vi "FTW-StressTest-Endpoint-CreateDestroy.vi"() -> ()   [LabVIEW 2012]
uses:
  src/Socket/FTW-Socket-Type.ctl
  src/Endpoint/FTW-Endpoint.lvclass
panel:
  out "x*y":i32
  out "error out":errorcluster
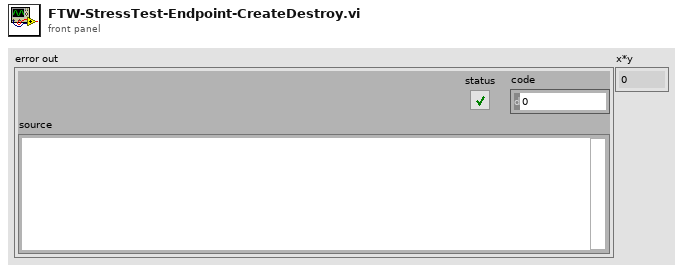
[diagram p1: front panel]
types:
  T1 = typedef "FTW-Actor.lvlib/FTW-Endpoint.lvclass/FTW-Socket-Type.ctl" = enum32{"NN_PAIR", "NN_PUB", "NN_SUB", "NN_REP", "NN_REQ", "NN_PUSH", "NN_PULL", "NN_SURVEYOR", "NN_RESPONDENT", "NN_BUS"}
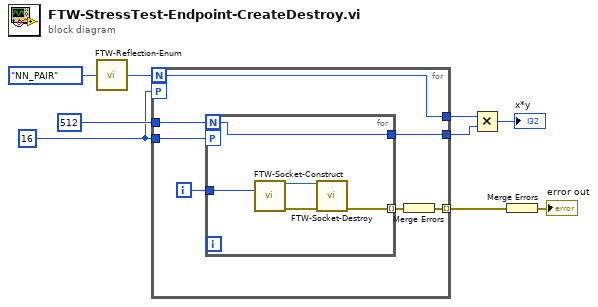
[diagram p0: block diagram]
diagram:
  w1 = 16
  n1 = call "FTW-Reflection-Enum.vi"("Enum"=FTW-Socket-Type."NN_PAIR" ("Socket Type")) -> ("Number of Items"=w5:i32)  [unwired: 12 in, 2 out]
  n2 = for {
    N: w5 -> [w11]
    tunnel: 512 -> [w16]
    tunnel: [w12] -> w8 mode=indexing
    tunnel: w1 -> [w15]
    tunnel: [w11] -> w4
    tunnel: [w10] -> w3
    workers-P: w1 -> [_]
    i -> [w14]
    n3 = for {
      N: w16 -> [w17]
      tunnel: [w18] -> w13 mode=indexing
      tunnel: w14 -> [w21]
      workers-P: w15 -> [_]
      tunnel: [w17] -> w10
      n4 = call "FTW-Socket-Construct.vi"("Socket Type"=w21) -> ("FTW Socket"=w19:refnum<class "FTW-Endpoint.lvclass">, "error out"=w20:errorcluster)  [unwired: 13 in]
      n5 = call-dynamic "FTW-Socket-Destroy.vi"("FTW Socket"=w19, "error in"=w20) -> ("error out"=w18:errorcluster)  [unwired: 13 in]
    }
    n6 = Merge Errors(w13) -> (w12:errorcluster)
  }
  n7 = Multiply(x=w4, y=w3) -> (x*y=→"x*y":i32)
  n8 = Merge Errors(w8) -> (→"error out":errorcluster)
